vi "NI-Embedded CAN for RIO subVI - CAN Frame to Table1.vi"(7 "Hexadecimal?":bool, 8 "error in (no error)":errorcluster, 9 "timestamp":timestamp, 10 "CAN frame":T1 {"type" items=["CAN Data", "CAN Remote"]; "identifier" format="%.0x"}, 11 "Input Array":string[][](array[string])) -> (3 "Output Array":string[][](array[string]), 4 "ilosc mesagy":dbl)   [LabVIEW 2015]
doc: "This example shows how to put a CAN transceiver to sleep on RIO Embedded CAN devices."
uses:
  <vilib>/RioEmbeddedCAN/RioEmbeddedCAN.llb/CANFrameControl.ctl
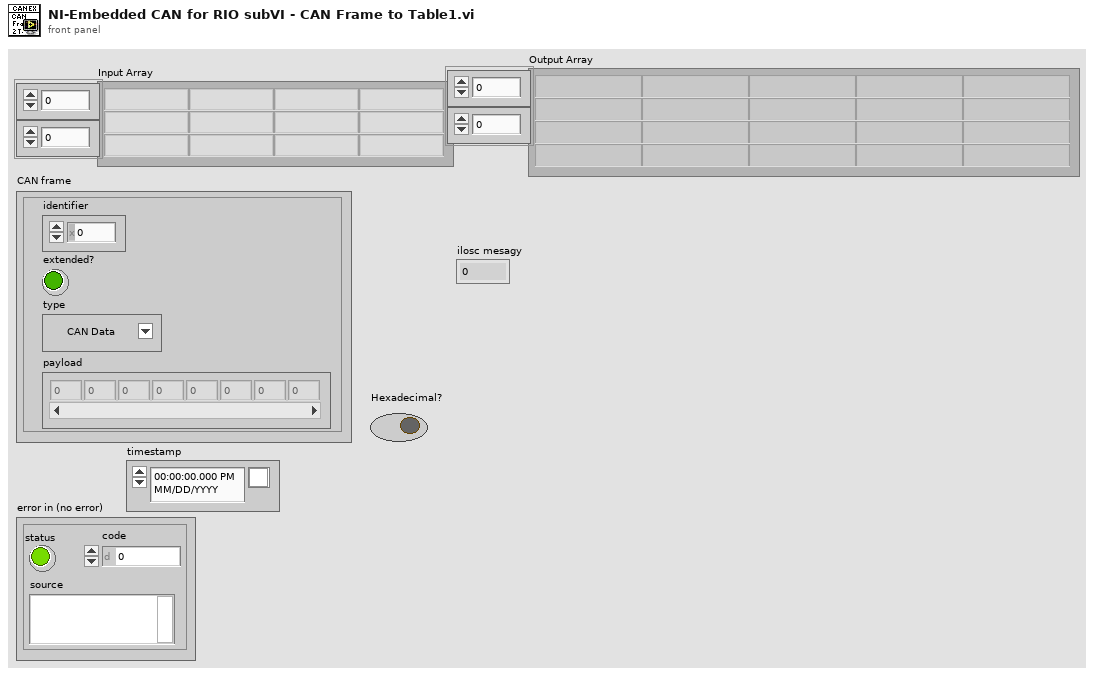
[diagram p1: front panel]
types:
  T1 = typedef "CANFrameControl.ctl" = cluster{"identifier":u32, "extended?":bool, "type":u8, "payload":u8[]}
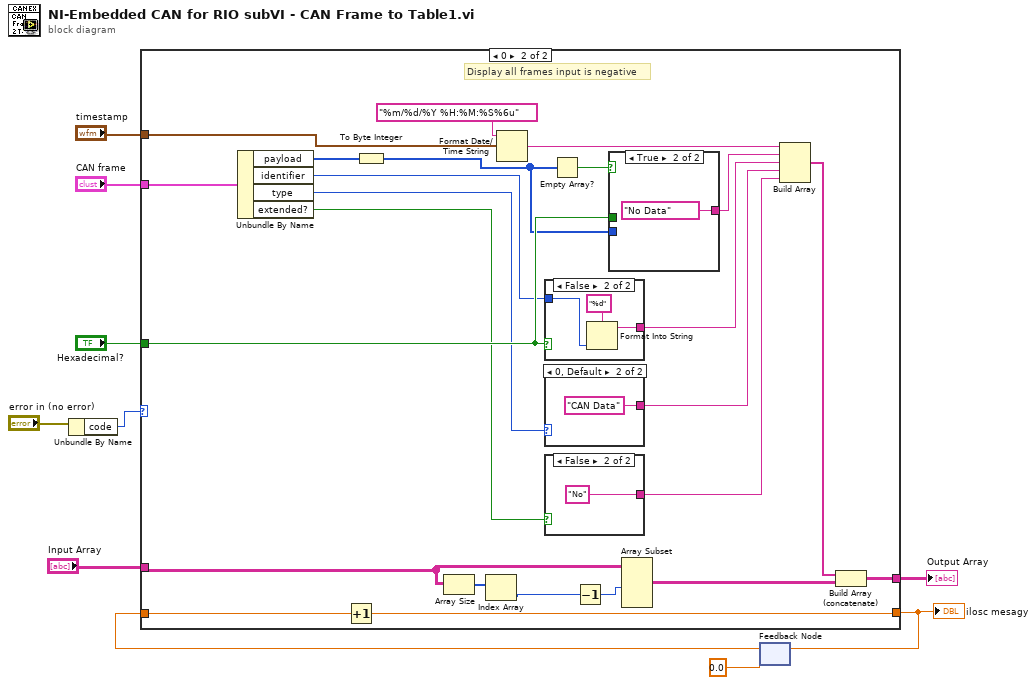
[diagram p0: block diagram]
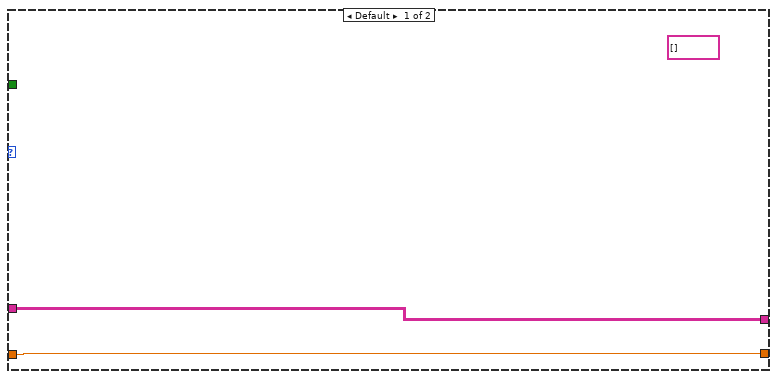
[diagram p2: hidden frame]
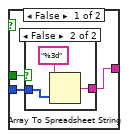
[diagram p3: hidden frame]
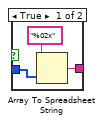
[diagram p4: hidden frame]
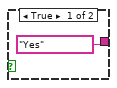
[diagram p5: hidden frame]
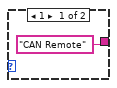
[diagram p6: hidden frame]
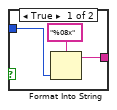
[diagram p7: hidden frame]
diagram:
  n1 = Unbundle By Name("error in (no error)") -> ("code"=w1:i32)
  n2 = feedback #1(0.0) -> (w4:dbl)
  n3 = case shown="0" w1 {
    tunnel: "Input Array" -> [w12 w35]
    tunnel: [w12 w34] -> w6
    tunnel: "Hexadecimal?" -> [_ w33]
    tunnel: "CAN frame" -> [_ w30]
    tunnel: "timestamp" -> [_ w15]
    tunnel: [w11 w32] -> w5
    tunnel: w4 -> [w11 w31]
    frame Default {
      (unwired) string[] []
    }
    frame 0 {
      # "Display all frames input is negative"
      n4 = Unbundle By Name(w30) -> ("payload"=w13:u8[], "identifier"=w16:u32, "type"=w23:u8, "extended?"=w20:bool)
      n5 = Increment(x=w31) -> (x+1=w32:dbl)
      n6 = To Byte Integer(number=w13) -> (8bit integer=w14:i8[])
      n7 = Array Size(array=w35) -> (size(s)=w36:i32[])
      n8 = Index Array(array=w36) -> (element=w28:i32)  [unwired: 1 in]
      n9 = Format Date/Time String(time format string (%c)="%m/%d/%Y %H:%M:%S%6u", seconds (now)=w15) -> (date/time string=w25:string)  [unwired: 1 in]
      n10 = case shown="False" w33 {
        tunnel: w16 -> [w52 w56]
        tunnel: [w51 w55] -> w24
        frame True {
          n11 = Format Into String(format string="%08x", w52) -> (resulting string=w51:string)  [unwired: 2 in, 1 out]
        }
        frame False {
          n12 = Format Into String(format string="%d", w56) -> (resulting string=w55:string)  [unwired: 2 in, 1 out]
        }
      }
      n13 = case shown="0, Default" w23 {
        tunnel: ["CAN Remote" "CAN Data"] -> w22
        frame 1 {
        }
        frame 0, Default {
        }
      }
      n14 = case shown="False" w20 {
        tunnel: ["Yes" "No"] -> w21
        frame True {
        }
        frame False {
        }
      }
      n15 = Empty Array?(array=w14) -> (empty?=w17:bool)
      n16 = Decrement(x=w28) -> (x-1=w29:i32)
      n17 = case shown="True" w17 {
        tunnel: [w37 "No Data"] -> w19
        tunnel: w14 -> [w39 _]
        tunnel: w33 -> [w38 _]
        frame False {
          n18 = case shown="False" w38 {
            tunnel: w39 -> [w40 w43]
            tunnel: [w41 w44] -> w37
            frame True {
              n19 = Array To Spreadsheet String(array=w40, 3:"%02x" ("format string")) -> (spreadsheet string=w41:string)  [unwired: 1 in]
            }
            frame False {
              n20 = Array To Spreadsheet String(array=w43, 3:"%3d" ("format string")) -> (spreadsheet string=w44:string)  [unwired: 1 in]
            }
          }
        }
        frame True {
        }
      }
      n21 = Array Subset(array=w35, length (row)=w29) -> (w26:string[][])  [unwired: 3 in]
      n22 = Build Array(w25, w19, w24, w22, w21) -> (w27:string[])
      n23 = Build Array (concatenate)(w27, w26) -> (w34:string[][])
    }
  }
  "Output Array" <- w6
  "ilosc mesagy" <- w5
  n24 = feedback-in #1(w5) -> ()
